vi "SetAuxIntakeSpeedDmd.vi"(11 "IntakeDemand":dbl) -> ()   [LabVIEW 2020]
uses:
  AuxGlobals.vi
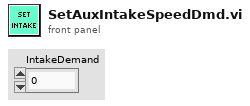
[diagram p1: front panel]
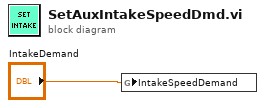
[diagram p0: block diagram]
diagram:
  n1 = global write "AuxGlobals.vi" "IntakeSpeedDemand"("IntakeDemand") -> ()
